vi "NanotecSMCPDDriver.VI-Tree.vi"   [LabVIEW 2015, in "NanotecSMCPDDriver.lvlib"]
doc: "This is the instrument driver for the Nanotec SMCI32, SMCI47, PD4-I and PD6-I controllers. The VI Tree displays all the user-callable VIs of the instrument driver in an organized table.\n\nFor more information and license information see the description of the containing thi s VI."
uses:
  NanotecSMCPDDriver.lvlib
panel:
  # "(c) 2006 <Enter Company Name Here>.  ALL RIGHTS RESERVED."
  # "SEE DIAGRAM\nFOR VI TREE."
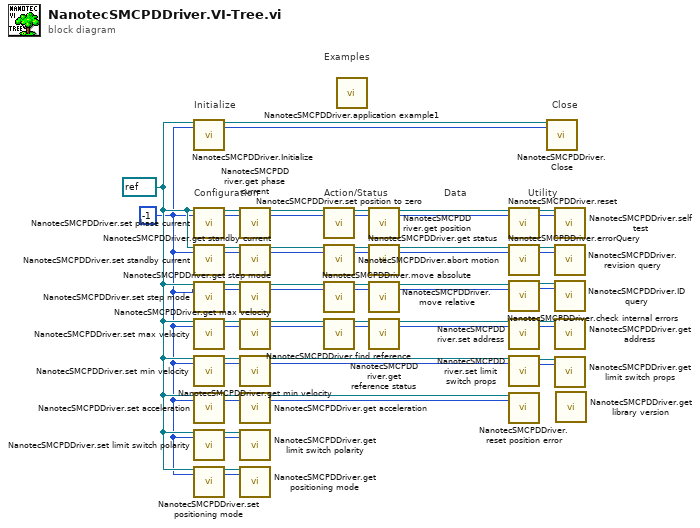
[diagram p0: block diagram]
diagram:
  w13 = refnum<visa-resource-name> refnum ("VISA resource name")
  w11 = -1 ("contollerID")
  # "Examples"
  # "Configuration"
  # "Utility"
  # "Data"
  # "Action/Status"
  # "Close"
  # "Initialize"
  n1 = call "NanotecSMCPDDriver.Initialize.vi"("VISA resource name"=w13, "contollerID"=w11) -> ("VISA resource name out"=w18:refnum<visa-resource-name>, "contollerID out"=w17:i32)  [unwired: 15 in, 1 out]
  n2 = call "NanotecSMCPDDriver.set phase current.vi"("VISA resource name"=w13, "contollerID"=w11) -> ("VISA resource name out"=w58:refnum<visa-resource-name>, "contollerID out"=w38:i32)  [unwired: 15 in, 1 out]
  n3 = call "NanotecSMCPDDriver.set standby current.vi"("VISA resource name"=w13, "contollerID"=w11) -> ("VISA resource name out"=w53:refnum<visa-resource-name>, "contollerID out"=w29:i32)  [unwired: 15 in, 1 out]
  n4 = call "NanotecSMCPDDriver.set step mode.vi"("VISA resource name"=w13, "contollerID"=w11) -> ("VISA resource name out"=w52:refnum<visa-resource-name>, "contollerID out"=w28:i32)  [unwired: 15 in, 1 out]
  n5 = call "NanotecSMCPDDriver.set max velocity.vi"("VISA resource name"=w13, "contollerID"=w11) -> ("VISA resource name out"=w51:refnum<visa-resource-name>, "contollerID out"=w21:i32)  [unwired: 15 in, 1 out]
  n6 = call "NanotecSMCPDDriver.set min velocity.vi"("VISA resource name"=w13, "contollerID"=w11) -> ("VISA resource name out"=w50:refnum<visa-resource-name>, "contollerID out"=w20:i32)  [unwired: 15 in, 1 out]
  n7 = call "NanotecSMCPDDriver.set acceleration.vi"("VISA resource name"=w13, "contollerID"=w11) -> ("VISA resource name out"=w49:refnum<visa-resource-name>, "contollerID out"=w19:i32)  [unwired: 15 in, 1 out]
  n8 = call "NanotecSMCPDDriver.set limit switch polarity.vi"("VISA resource name"=w13, "contollerID"=w11) -> ("VISA resource name out"=w16:refnum<visa-resource-name>, "contollerID out"=w15:i32)  [unwired: 15 in, 1 out]
  n9 = call "NanotecSMCPDDriver.set positioning mode.vi"("VISA resource name"=w13, "contollerID"=w11) -> ("VISA resource name out"=w14:refnum<visa-resource-name>, "contollerID out"=w12:i32)  [unwired: 15 in, 1 out]
  n10 = call "NanotecSMCPDDriver.get phase current.vi"("VISA resource name"=w58, "contollerID"=w38) -> ("VISA resource name out"=w57:refnum<visa-resource-name>, "contollerID out"=w37:i32)  [unwired: 14 in, 2 out]
  n11 = call "NanotecSMCPDDriver.get standby current.vi"("VISA resource name"=w53, "contollerID"=w29) -> ("VISA resource name out"=w46:refnum<visa-resource-name>, "contollerID out"=w30:i32)  [unwired: 14 in, 2 out]
  n12 = call "NanotecSMCPDDriver.get step mode.vi"("VISA resource name"=w52, "contollerID"=w28) -> ("VISA resource name out"=w47:refnum<visa-resource-name>, "contollerID out"=w27:i32)  [unwired: 14 in, 2 out]
  n13 = call "NanotecSMCPDDriver.get max velocity.vi"("VISA resource name"=w51, "contollerID"=w21) -> ("VISA resource name out"=w48:refnum<visa-resource-name>, "contollerID out"=w22:i32)  [unwired: 14 in, 2 out]
  n14 = call "NanotecSMCPDDriver.get min velocity.vi"("VISA resource name"=w50, "contollerID"=w20) -> ("VISA resource name out"=w10:refnum<visa-resource-name>, "contollerID out"=w7:i32)  [unwired: 14 in, 2 out]
  n15 = call "NanotecSMCPDDriver.get acceleration.vi"("VISA resource name"=w49, "contollerID"=w19) -> ("VISA resource name out"=w6:refnum<visa-resource-name>, "contollerID out"=w5:i32)  [unwired: 14 in, 2 out]
  n16 = call "NanotecSMCPDDriver.get limit switch polarity.vi"("VISA resource name"=w16, "contollerID"=w15) -> ()  [unwired: 14 in, 4 out]
  n17 = call "NanotecSMCPDDriver.get positioning mode.vi"("VISA resource name"=w14, "contollerID"=w12) -> ()  [unwired: 14 in, 4 out]
  n18 = call "NanotecSMCPDDriver.set position to zero.vi"("VISA resource name"=w57, "contollerID"=w37) -> ("VISA resource name out"=w56:refnum<visa-resource-name>, "contollerID out"=w36:i32)  [unwired: 15 in, 1 out]
  n19 = call "NanotecSMCPDDriver.abort motion.vi"("VISA resource name"=w46, "contollerID"=w30) -> ("VISA resource name out"=w45:refnum<visa-resource-name>, "contollerID out"=w31:i32)  [unwired: 15 in, 1 out]
  n20 = call "NanotecSMCPDDriver.move absolute.vi"("VISA resource name"=w47, "contollerID"=w27) -> ("VISA resource name out"=w44:refnum<visa-resource-name>, "contollerID out"=w26:i32)  [unwired: 15 in, 1 out]
  n21 = call "NanotecSMCPDDriver.find reference.vi"("VISA resource name"=w48, "contollerID"=w22) -> ("VISA resource name out"=w4:refnum<visa-resource-name>, "contollerID out"=w2:i32)  [unwired: 15 in, 1 out]
  n22 = call "NanotecSMCPDDriver.application example1.vi"() -> ()  [unwired: 1 in]
  n23 = call "NanotecSMCPDDriver.get position.vi"("VISA resource name"=w56, "contollerID"=w36) -> ("VISA resource name out"=w55:refnum<visa-resource-name>, "contollerID out"=w35:i32)  [unwired: 14 in, 2 out]
  n24 = call "NanotecSMCPDDriver.get status.vi"("VISA resource name"=w45, "contollerID"=w31) -> ("VISA resource name out"=w42:refnum<visa-resource-name>, "contollerID out"=w32:i32)  [unwired: 14 in, 2 out]
  n25 = call "NanotecSMCPDDriver.move relative.vi"("VISA resource name"=w44, "contollerID"=w26) -> ("VISA resource name out"=w43:refnum<visa-resource-name>, "contollerID out"=w25:i32)  [unwired: 15 in, 1 out]
  n26 = call "NanotecSMCPDDriver.get reference status.vi"("VISA resource name"=w4, "contollerID"=w2) -> ("VISA resource name out"=w3:refnum<visa-resource-name>, "contollerID out"=w1:i32)  [unwired: 15 in, 1 out]
  n27 = call "NanotecSMCPDDriver.reset.vi"("VISA resource name"=w55, "contollerID"=w35) -> ("VISA resource name out"=w54:refnum<visa-resource-name>, "contollerID out"=w34:i32)  [unwired: 15 in, 1 out]
  n28 = call "NanotecSMCPDDriver.errorQuery.vi"("VISA resource name"=w42, "contollerID"=w32) -> ("VISA resource name out"=w41:refnum<visa-resource-name>, "contollerID out"=w33:i32)  [unwired: 13 in, 3 out]
  n29 = call "NanotecSMCPDDriver.check internal errors.vi"("VISA resource name"=w43, "contollerID"=w25) -> ("VISA resource name out"=w40:refnum<visa-resource-name>, "contollerID out"=w24:i32)  [unwired: 13 in, 3 out]
  n30 = call "NanotecSMCPDDriver.set address.vi"("VISA resource name"=w3, "contollerID"=w1) -> ("VISA resource name out"=w39:refnum<visa-resource-name>, "contollerID out"=w23:i32)  [unwired: 15 in, 1 out]
  n31 = call "NanotecSMCPDDriver.set limit switch props.vi"("VISA resource name"=w10, "contollerID"=w7) -> ("VISA resource name out"=w9:refnum<visa-resource-name>, "contollerID out"=w8:i32)  [unwired: 15 in, 1 out]
  n32 = call "NanotecSMCPDDriver.reset position error.vi"("VISA resource name"=w6, "contollerID"=w5) -> ()  [unwired: 15 in, 3 out]
  n33 = call "NanotecSMCPDDriver.Close.vi"("VISA resource name"=w18, "contollerID"=w17) -> ()  [unwired: 17 in, 1 out]
  n34 = call "NanotecSMCPDDriver.self test.vi"("VISA resource name"=w54, "contollerID"=w34) -> ()  [unwired: 13 in, 5 out]
  n35 = call "NanotecSMCPDDriver.revision query.vi"("VISA resource name"=w41, "contollerID"=w33) -> ()  [unwired: 13 in, 5 out]
  n36 = call "NanotecSMCPDDriver.ID query.vi"("VISA resource name"=w40, "contollerID"=w24) -> ()  [unwired: 13 in, 5 out]
  n37 = call "NanotecSMCPDDriver.get address.vi"("VISA resource name"=w39, "contollerID"=w23) -> ()  [unwired: 14 in, 4 out]
  n38 = call "NanotecSMCPDDriver.get limit switch props.vi"("VISA resource name"=w9, "contollerID"=w8) -> ()  [unwired: 14 in, 4 out]
  n39 = call "NanotecSMCPDDriver.get library version.vi"() -> ()  [unwired: 1 in, 1 out]
